vi "calculate_scanner_delays_own.vi"(8 "error in (no error)":errorcluster, 9 "position feedback data":T2, 10 "transformation parameters":T1={"scale factor"=1.0, "rotation angle"=0.0, "tilting angle"=0.0, "offset"=refnum}, 11 "TrajectoryDL090201FrameScan in":refnum<class "TrajectoryDL090201FrameScan.lvclass">) -> (0 "error out":errorcluster, 3 "TrajectoryDL090201FrameScan out":refnum<class "TrajectoryDL090201FrameScan.lvclass">)   [LabVIEW 2010, in "TrajectoryDL090201FrameScan.lvclass"]
uses:
  TrajectoryDL090201FrameScan.lvclass
  common/arrays/pixel_raw_data_array.ctl
  TrajectoryDL091126GenericVoxel/TrajectoryDL091126GenericVoxel/transformation_parameters.ctl
  common/classes/SpaceVector/SpaceVector/SpaceVector.lvclass
  common/classes/ErrorController/ErrorController/class_data.vi
  TrajectoryDL091126GenericVoxel/TrajectoryDL091126GenericVoxel/TrajectoryDL091126GenericVoxel.lvclass
  <vilib>/Analysis/NI_AALPro.lvlib
  common/classes/ErrorController/ErrorController/ErrorController.lvclass
panel:
  out "x position feedback signal and 2nd derivative 2":dbl[unit][][](graph)
  out "x position feedback signal and 2nd derivative":dbl[][](graph)
  out "z position feedback signal and 2nd derivative":dbl[][](graph)
  out "y position feedback signal and 2nd derivative":dbl[][](graph)
  out "calculated scanner delays":i32[](array[numeric])
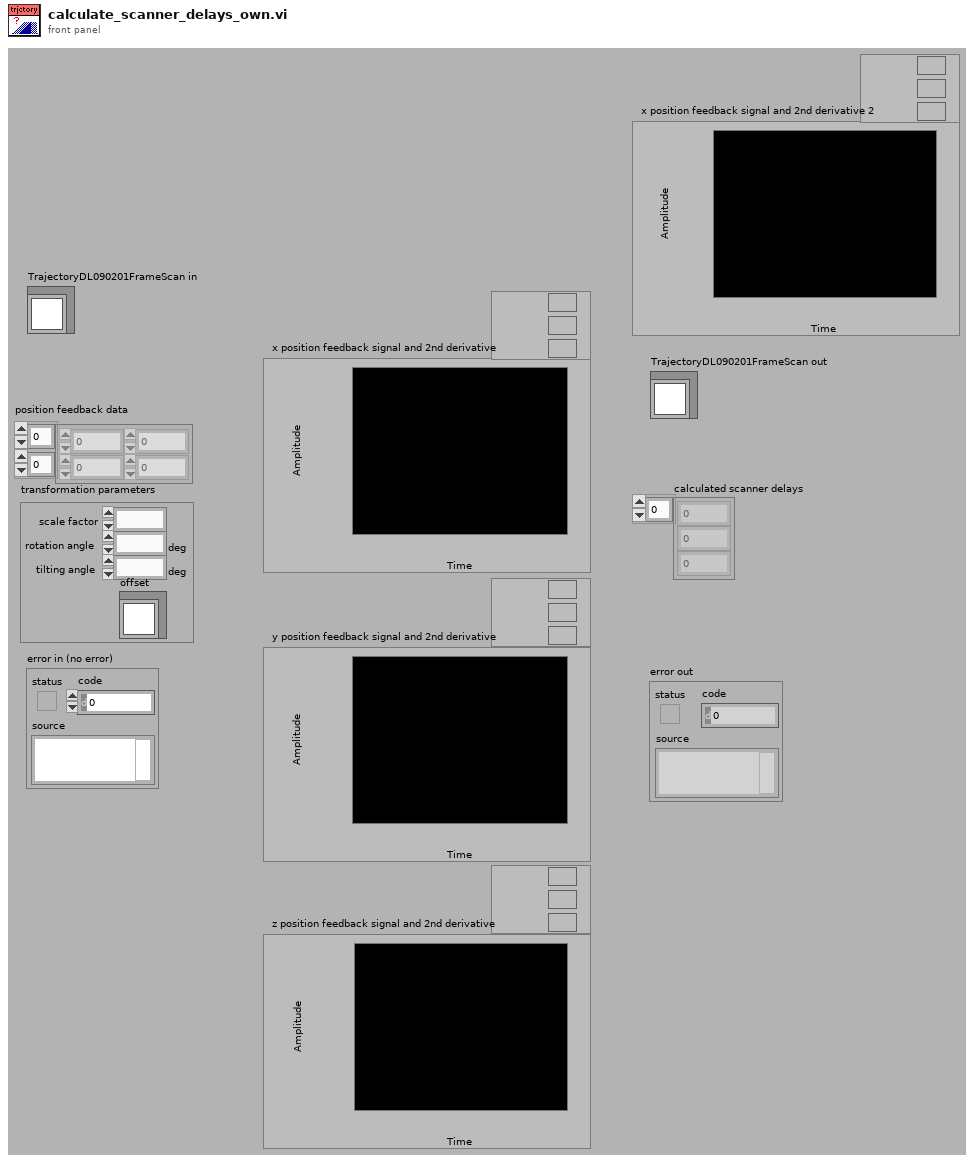
[diagram p1: front panel]
types:
  T1 = typedef "TrajectoryDL091126GenericVoxel.lvclass/transformation_parameters.ctl" = cluster{"scale factor":dbl, "rotation angle":dbl[unit], "tilting angle":dbl[unit], "offset":refnum<class "SpaceVector.lvclass">}
  T2 = typedef "pixel_raw_data_array.ctl" = dbl[][]
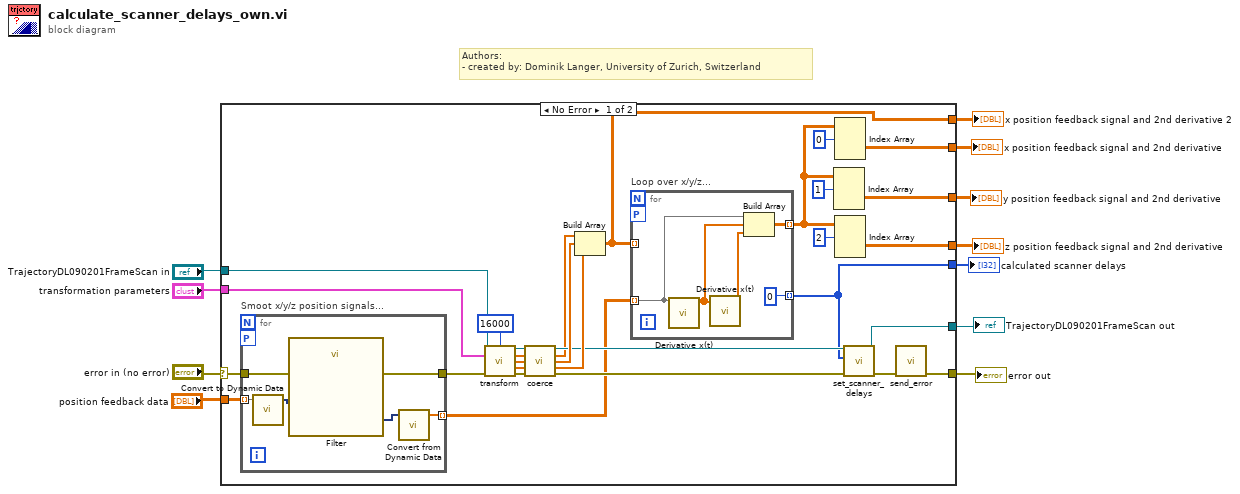
[diagram p0: block diagram]
diagram:
  # "Authors: \n- created by: Dominik Langer, University of Zurich, Switzerland"
  n1 = case shown="No Error" "error in (no error)" {
    selector: "error in (no error)" -> [w18 w53]
    tunnel: [w12 w53] -> w6
    tunnel: [w27 w52] -> w7
    tunnel: [w28 _] -> w5
    tunnel: "position feedback data" -> [w17 _]
    tunnel: "TrajectoryDL090201FrameScan in" -> [w38 w52]
    tunnel: "transformation parameters" -> [w40 _]
    tunnel: [w25 _] -> w4
    tunnel: [w24 _] -> w3
    tunnel: [w23 _] -> w2
    tunnel: [w14 _] -> w1
    frame No Error {
      n2 = for "Smoot x/y/z position signals..." {
        tunnel: [w41] -> w15 mode=indexing
        tunnel: w18 -> [w45]
        tunnel: w17 -> [w44] mode=indexing
        workers-P: _ -> [_]
        tunnel: [w43] -> w16
        n3 = call "Convert to Dynamic Data"("Array"=w44) -> ("Dynamic Data Type"=w46:dynamicdata)  [unwired: 3 in]
        n4 = call "Filter"("error in (no error)"=w45, "Signal"=w46) -> ("error out"=w43:errorcluster, "Filtered Signal"=w42:dynamicdata)  [unwired: 8 in]
        n5 = call "Convert from Dynamic Data"("Dynamic Data Type"=w42) -> ("Array"=w41:dbl[])  [unwired: 3 in]
      }
      n6 = call-dynamic "transform.vi"("GenericTrajectory in"=w38, "number of pixels (all: -1)"=16000, "transformation parameters"=w40, "error in (no error)"=w16) -> ("GenericTrajectory out"=w39:refnum<class "TrajectoryDL090201FrameScan.lvclass">, "x coordinates"=w36:dbl[unit][], "y coordinates"=w35:dbl[unit][], "z coordinates"=w34:dbl[unit][], "error out"=w37:errorcluster)  [unwired: 7 in]
      n7 = call "coerce.vi"("GenericTrajectory in"=w39, "x coordinates in"=w36, "y coordinates in"=w35, "z coordinates in"=w34, "error in (no error)"=w37) -> ("GenericTrajectory out"=w29:refnum<class "TrajectoryDL090201FrameScan.lvclass">, "x coordinates out"=w19:dbl[unit][], "y coordinates out"=w33:dbl[unit][], "z coordinates out"=w32:dbl[unit][], "error out"=w30:errorcluster)  [unwired: 5 in, 1 out]
      n8 = Build Array(w19, w33, w32) -> (w14:dbl[unit][][])
      n9 = for "Loop over x/y/z..." {
        tunnel: w15 -> [w47] mode=indexing
        tunnel: [0] -> w28 mode=indexing
        workers-P: _ -> [_]
        tunnel: [w50] -> w26 mode=indexing
        tunnel: w14 -> [_] mode=indexing
        n10 = call <vilib>:"Derivative x(t).vi"("X"=w47) -> ("dX/dt"=w48:dbl[])  [unwired: 9 in, 1 out]
        n11 = call <vilib>:"Derivative x(t).vi"("X"=w48) -> ("dX/dt"=w49:dbl[])  [unwired: 9 in, 1 out]
        n12 = Build Array(w47, w48, w49) -> (w50:dbl[][])
      }
      n13 = Index Array(array=w26, index (dim 0)=1 ("index (page)")) -> (element=w24:dbl[][])  [unwired: 2 in]
      n14 = Index Array(array=w26, index (dim 0)=0 ("index (page)")) -> (element=w25:dbl[][])  [unwired: 2 in]
      n15 = Index Array(array=w26, index (dim 0)=2 ("index (page)")) -> (element=w23:dbl[][])  [unwired: 2 in]
      n16 = call-dynamic "set_scanner_delays.vi"("error in (no error)"=w30, "scanner delays"=w28, "TrajectoryDL091126GenericVoxel in"=w29) -> ("error out"=w13:errorcluster, "TrajectoryDL091126GenericVoxel out"=w27:refnum<class "TrajectoryDL090201FrameScan.lvclass">)  [unwired: 7 in]
      n17 = call "send_error.vi"("error in (no error)"=w13) -> ("error out"=w12:errorcluster)  [unwired: 10 in]
    }
    frame Error {
    }
  }
  "error out" <- w6
  "TrajectoryDL090201FrameScan out" <- w7
  "calculated scanner delays" <- w5
  "y position feedback signal and 2nd derivative" <- w3
  "z position feedback signal and 2nd derivative" <- w2
  "x position feedback signal and 2nd derivative" <- w4
  "x position feedback signal and 2nd derivative 2" <- w1
